vi "Unflatten From JSON.vi"() -> ()   [LabVIEW 2023]
doc: "Demonstrates the LabVIEW JSON (JavaScript Object Notation) parser by flattening a cluster to JSON then unflattening it back into multiple pieces."
uses:
  <vilib>/silver_ctls/ArrayMatrixCluster/Real Matrix NI_Silver.ctl
  JSON_Example_Input.ctl
panel:
  out "Remaining Unflattened Data":T1
  out "Unflattened Error":errorcluster
  out "Unflattened Cell":dbl
  out "Unflattened First Data Row":dbl[](array[numeric])
  out "Unflattened Time":timestamp
  out "Unflattened Name":string
  out "JSON":string
  in  "Input":T2={"Description"={"Name"="Test Data", "Time"=0}, "Data"=[[-1.0, 0.0, -1.0, 0.0], [1.0, 0.25, 0.0, 0.75], [-0.5, 0.0, 1.0, 0.0]], "Error"={"status"=TRUE, "code"=1, "source"="Testing"}}
  # "Overview: Demonstrates the LabVIEW JSON (JavaScript Object Notation) parser by flattening a cluster to JSON then unflattening it back into multiple pieces. The JSON output will be encoded in UTF-8, which may not correctly display on some systems.\nInstructions:\nRun the VI."
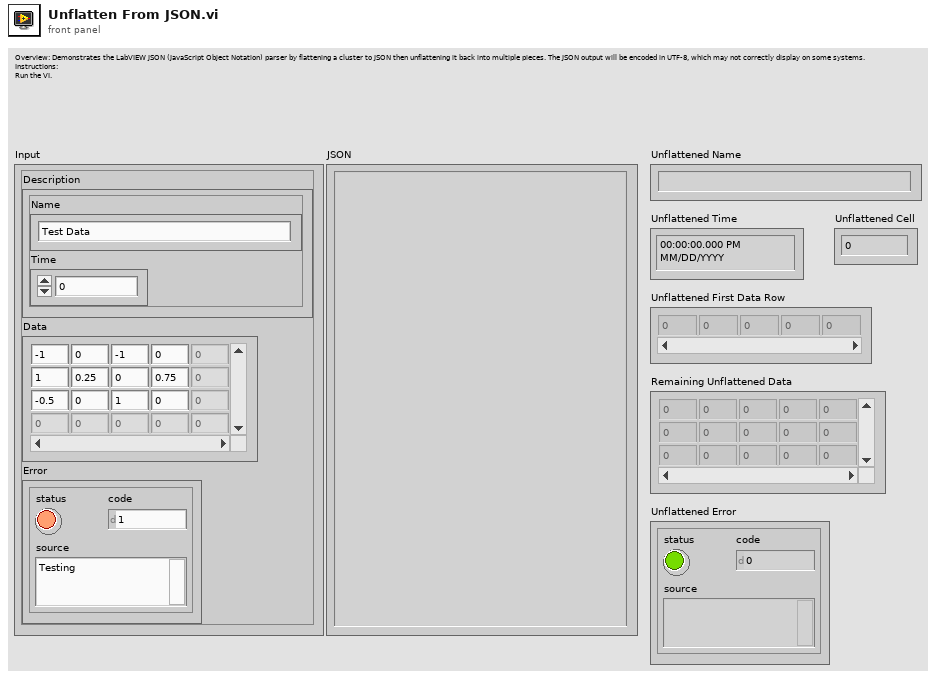
[diagram p1: front panel]
types:
  T1 = typedef "Real Matrix NI_Silver.ctl" = dbl[][]
  T2 = cluster{"Description":cluster{"Name":string, "Time":u64}, "Data":T1, "Error":errorcluster}
  T3 = typedef "JSON_Example_Input.ctl" = cluster{"Description":cluster{"Name":string, "Time":u64}, "Data":T1, "Error":errorcluster}
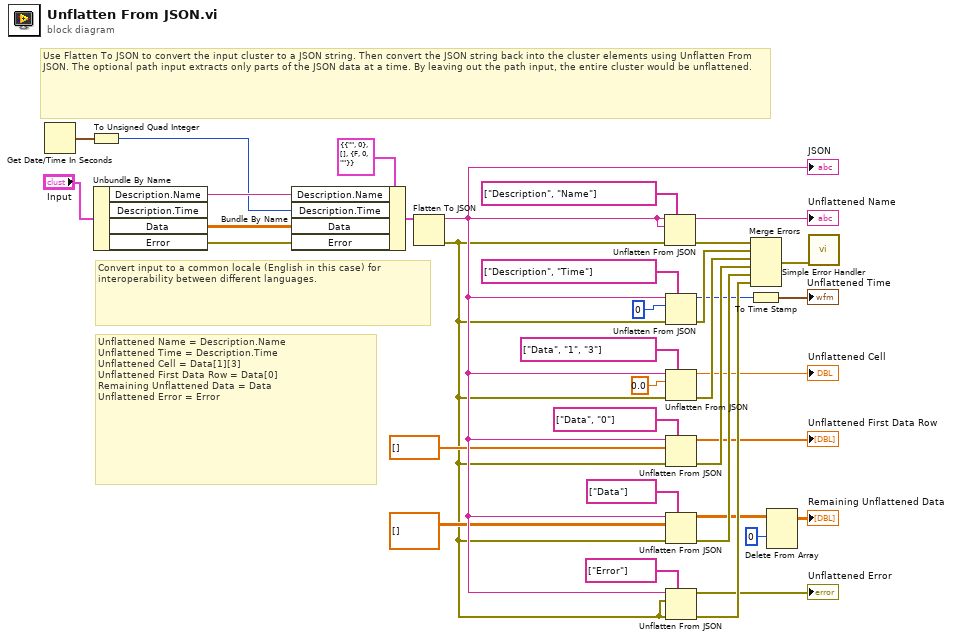
[diagram p0: block diagram]
diagram:
  # "Convert input to a common locale (English in this case) for interoperability between different languages."
  # "Unflattened Name = Description.Name\nUnflattened Time = Description.Time\nUnflattened Cell = Data[1][3]\nUnflattened First Data Row = Data[0]\nRemaining Unflattened Data = Data\nUnflattened Error = Error"
  # "Use Flatten To JSON to convert the input cluster to a JSON string. Then convert the JSON string back into the cluster elements using Unflatten From JSON. The optional path input extracts only parts of the JSON data at a time. By leaving out the path input, the entire cluster would be unflattened."
  n1 = Get Date/Time In Seconds() -> (seconds since 1Jan1904=w36:timestamp)
  n2 = To Unsigned Quad Integer(1:w36) -> (0:w3:u64)
  n3 = Unbundle By Name("Input") -> ("Description.Name"=w6:string, "Data"=w5:T1, "Error"=w4:errorcluster)  [unwired: 1 out]
  n4 = Bundle By Name(cluster=T3 {"Description"={"Name"="", "Time"=0}, "Data"=[], "Error"={"status"=FALSE, "code"=0, "source"=""}} ("Input"), "Description.Name"=w6, "Description.Time"=w3, "Data"=w5, "Error"=w4) -> (w35:T3)
  n5 = Flatten To JSON(anything=w35) -> (JSON string=w18:string, 11:w8:errorcluster)  [unwired: 2 in]
  "JSON" <- w18
  n6 = Unflatten From JSON(path=string[] ["Description", "Name"], JSON string=w18, type and defaults=w18, error in (no error)=w8) -> (value=→"Unflattened Name":string, error out=w34:errorcluster)  [unwired: 3 in]
  n7 = Unflatten From JSON(path=string[] ["Description", "Time"], JSON string=w18, type and defaults=u64 0, error in (no error)=w8) -> (value=w19:u64, error out=w30:errorcluster)  [unwired: 3 in]
  n8 = Unflatten From JSON(path=string[] ["Data", "1", "3"], JSON string=w18, type and defaults=0.0, error in (no error)=w8) -> (value=→"Unflattened Cell":dbl, error out=w29:errorcluster)  [unwired: 3 in]
  n9 = Unflatten From JSON(path=string[] ["Data", "0"], JSON string=w18, type and defaults=dbl[] [], error in (no error)=w8) -> (value=→"Unflattened First Data Row":dbl[], error out=w28:errorcluster)  [unwired: 3 in]
  n10 = Unflatten From JSON(path=string[] ["Data"], JSON string=w18, type and defaults=T1 [] ("Remaining Unflattened Data"), error in (no error)=w8) -> (value=w22:T1, error out=w27:errorcluster)  [unwired: 3 in]
  n11 = Unflatten From JSON(path=string[] ["Error"], JSON string=w18, type and defaults=w8, error in (no error)=w8) -> (value=→"Unflattened Error":errorcluster, error out=w24:errorcluster)  [unwired: 3 in]
  n12 = Merge Errors(w34, w30, w29, w28, w27, w24) -> (w31:errorcluster)
  n13 = To Time Stamp(1:w19) -> (0:→"Unflattened Time":timestamp)
  n14 = Delete From Array(array=w22, index (row)=0) -> (array with subset deleted=→"Remaining Unflattened Data":T1)  [unwired: 2 in, 1 out]
  n15 = call <vilib>:"Simple Error Handler.vi"("error in (no error)"=w31) -> ()  [unwired: 4 in, 5 out]
